vi "Read Value.vi"(8 "error in (no error)":errorcluster, 11 "WriteAnalog in":refnum<class "WriteAnalog.lvclass">) -> (0 "error out":errorcluster, 2 "Value":u16 max=4095, 3 "WriteAnalog out":refnum<class "WriteAnalog.lvclass">)   [LabVIEW 2013, in "HardwareCharacterization.lvlib" / "WriteAnalog.lvclass"]
uses:
  WriteAnalog.lvclass
  WriteAnalog.lvclass/WriteAnalog.ctl
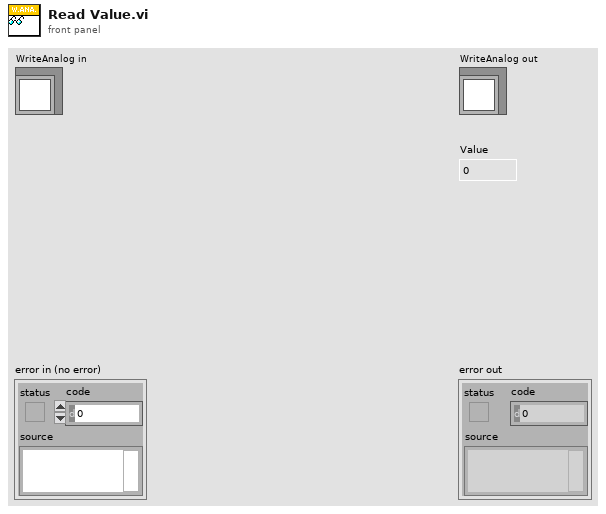
[diagram p1: front panel]
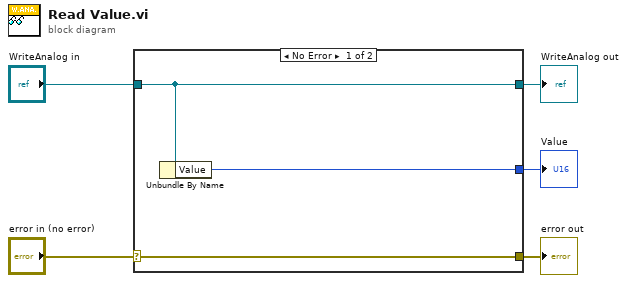
[diagram p0: block diagram]
diagram:
  n1 = case shown="No Error" "error in (no error)" {
    selector: "error in (no error)" -> [w8 w9]
    tunnel: [w8 w9] -> w4
    tunnel: [w7 w10] -> w2
    tunnel: "WriteAnalog in" -> [w7 w10]
    tunnel: [w6 _] -> w1
    frame No Error {
      n2 = Unbundle By Name(w7) -> ("Value"=w6:u16)
    }
    frame Error {
    }
  }
  "error out" <- w4
  "WriteAnalog out" <- w2
  "Value" <- w1
